vi "AMZ_S3_APIHLP_Parse DateTime String to TimeStamp.vi"(8 "error in (no error)":errorcluster, 11 "DateTime String":string) -> (0 "error out":errorcluster, 3 "Time Stamp":timestamp)   [LabVIEW 2015, in "LV Interface for Amazon S3.lvlib"]
doc: "Parses a DateTime string returned by Amazon S3 to a LV Time Stamp."
uses:
  LV Interface for Amazon S3.lvlib
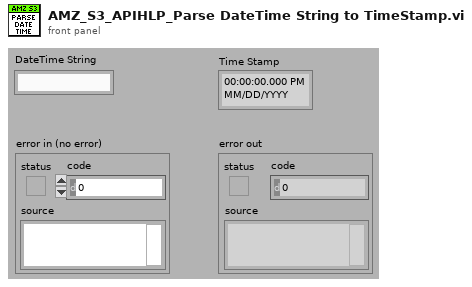
[diagram p1: front panel]
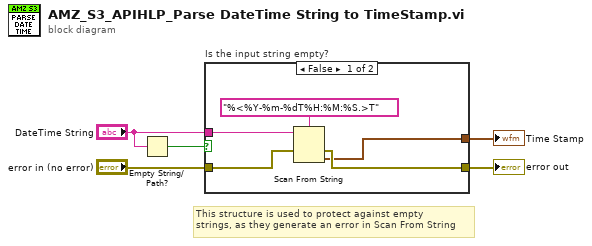
[diagram p0: block diagram]
diagram:
  # "This structure is used to protect against empty\nstrings, as they generate an error in Scan From String"
  n1 = Empty String/Path?(string/path="DateTime String") -> (empty?=w5:bool)
  n2 = case "Is the input string empty?" shown="False" w5 {
    tunnel: "DateTime String" -> [w9 _]
    tunnel: "error in (no error)" -> [w8 w11]
    tunnel: [w7 w11] -> w2
    tunnel: [w6 _] -> w1
    frame False {
      n3 = Scan From String(format string="%<%Y-%m-%dT%H:%M:%S.>T", input string=w9, error in=w8) -> (error out=w7:errorcluster, output 1=w6:timestamp)  [unwired: 2 in, 2 out]
    }
    frame True {
    }
  }
  "Time Stamp" <- w1
  "error out" <- w2
